vi "Conversao_valores_UCM.0200_SAIDA.vi"(11 "UCM.004.EEL.0200_SAIDA(Controle)":T1) -> (3 "UCM.004.EEL.0200_SAIDA(Indicador)":T1)   [LabVIEW 2019]
uses:
  padrao_UCM.004.EEL.0200_SAIDA.ctl
panel:
  in  "ANALOGICO_saida":cluster{"GD-ST-ES":i16, "X33-2":i16}
  out "ANALOGICO_entrada":cluster{"GD-ST-ES":i16, "X33-2":i16}
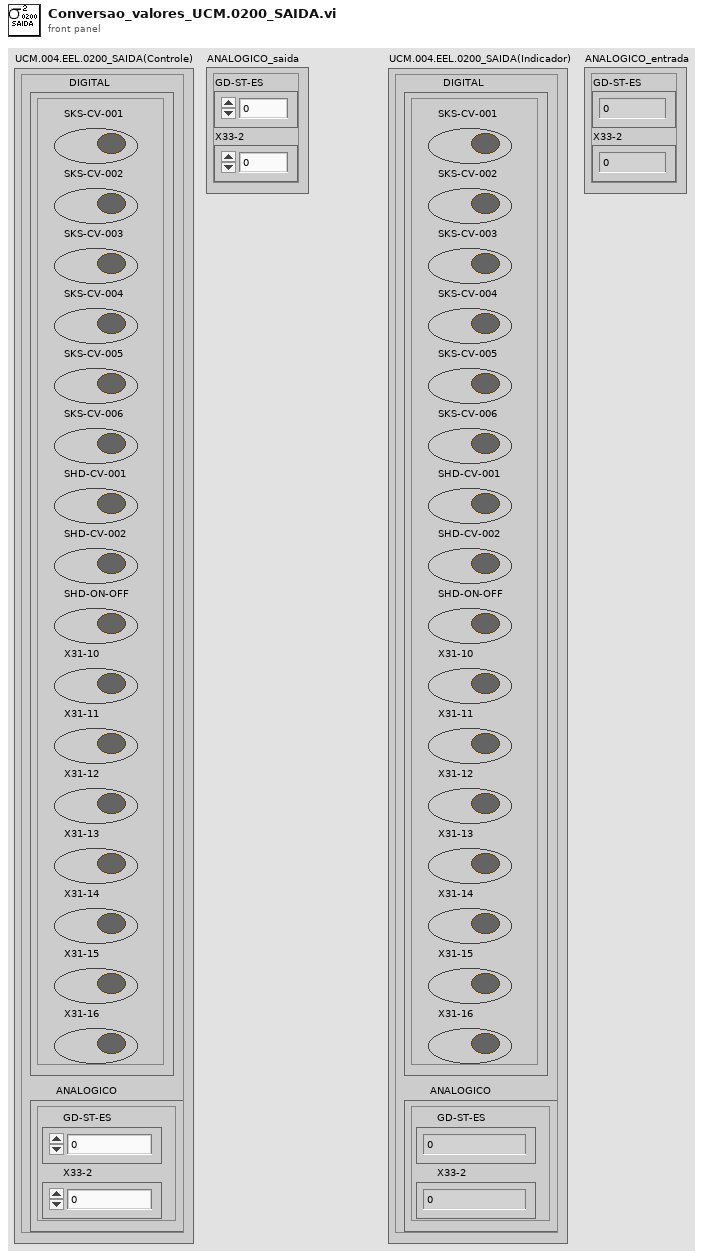
[diagram p1: front panel]
types:
  T1 = typedef "padrao_UCM.004.EEL.0200_SAIDA.ctl" = cluster{"DIGITAL":cluster{"SKS-CV-001":bool, "SKS-CV-002":bool, "SKS-CV-003":bool, "SKS-CV-004":bool, "SKS-CV-005":bool, "SKS-CV-006":bool, "SHD-CV-001":bool, "SHD-CV-002":bool, "SHD-ON-OFF":bool, "X31-10":bool, "X31-11":bool, "X31-12":bool, "X31-13":bool, "X31-14":bool, "X31-15":bool, "X31-16":bool}, "ANALOGICO":cluster{"GD-ST-ES":i16, "X33-2":i16}}
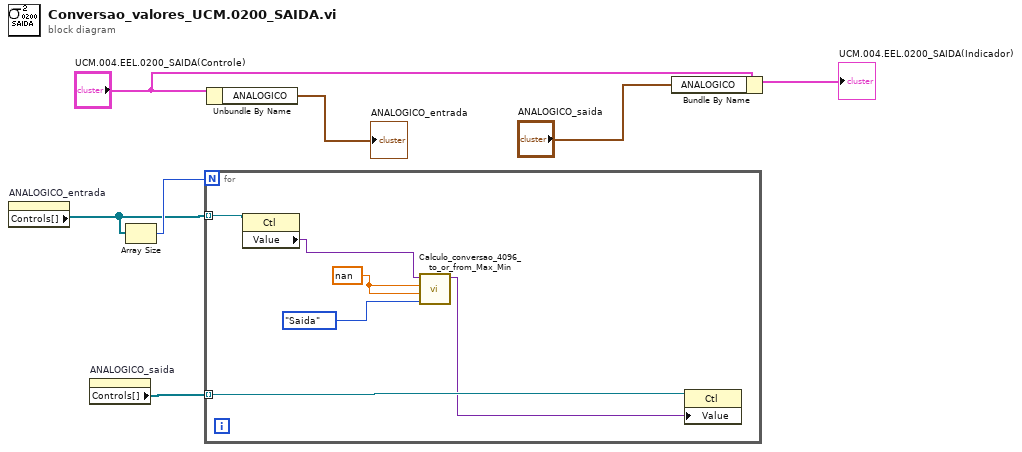
[diagram p0: block diagram]
diagram:
  n1 = property on="ANALOGICO_entrada" class="Clust (strict)"() -> ("Controls[]"=w2:refnum<vi>[])  [unwired: 2 in, 2 out]
  n2 = property on="ANALOGICO_saida" class="Clust (strict)"() -> ("Controls[]"=w1:refnum<vi>[])  [unwired: 2 in, 2 out]
  n3 = Array Size(array=w2) -> (size(s)=w7:i32)
  n4 = for {
    N: w7 -> [_]
    tunnel: w2 -> [w9] mode=indexing
    tunnel: w1 -> [w13] mode=indexing
    w11 = nan
    n5 = property class="Ctl"(reference=w9) -> ("Value"=w8:variant)  [unwired: 1 in, 2 out]
    n6 = call "Calculo_conversao_4096_to_or_from_Max_Min.vi"("Tipo"=enum16{"Saida", "Entrada"}."Saida", "Min"=w11, "Max"=w11, "Value"=w8) -> ("Value 2"=w10:variant)  [unwired: 7 in]
    n7 = property class="Ctl"(reference=w13, "Value"=w10) -> ()  [unwired: 1 in, 2 out]
  }
  n8 = Unbundle By Name("UCM.004.EEL.0200_SAIDA(Controle)") -> ("ANALOGICO"=→"ANALOGICO_entrada":cluster{"GD-ST-ES":i16, "X33-2":i16})
  n9 = Bundle By Name(cluster="UCM.004.EEL.0200_SAIDA(Controle)", "ANALOGICO"="ANALOGICO_saida") -> (→"UCM.004.EEL.0200_SAIDA(Indicador)":T1)
